vi "FRC.vi"(0 "System no.":i32=1 min=1 max=4 step=1, 1 "Base routine name":string, 2 "Routines to couple to":string[](array[string]), 4 "Remove routine coupling?":bool, 5 "error in":errorcluster) -> (19 "error out":errorcluster)   [LabVIEW 2020]
doc: "Set fast alignment routine coupling: \nIf coupling should be removed, \"Routines to couple to\" has to be 0 or \"Remove routine coupling\" has to be TRUE.\n\nC-887, E-712:"
panel:
  # "Sets Fast alignment Routine Coupling."
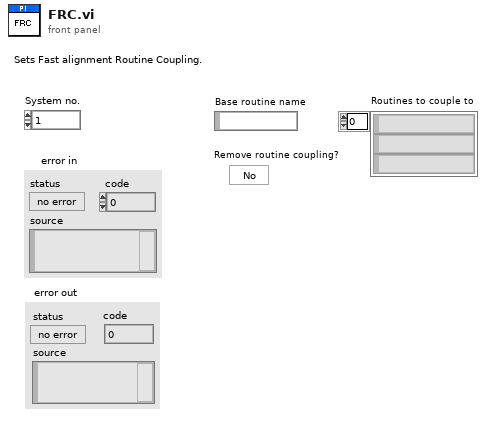
[diagram p1: front panel]
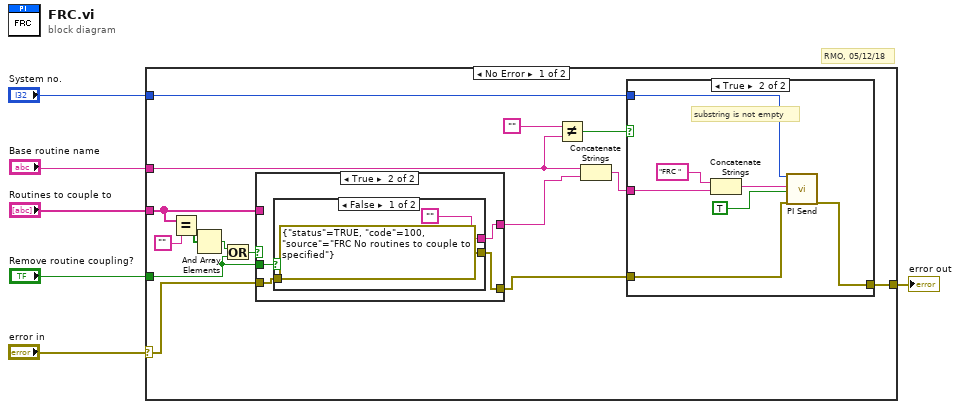
[diagram p0: block diagram]
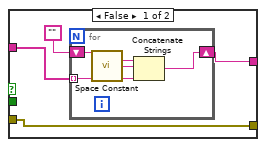
[diagram p2: hidden frame]
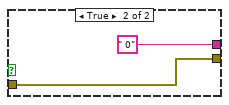
[diagram p3: hidden frame]
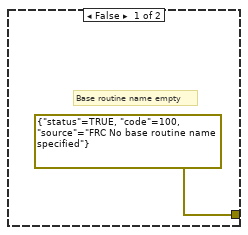
[diagram p4: hidden frame]
diagram:
  # "RMO, 05/12/18"
  n1 = case shown="No Error" "error in" {
    selector: "error in" -> [w7 w46]
    tunnel: [w21 w46] -> w6
    tunnel: "System no." -> [w20 _]
    tunnel: "Base routine name" -> [w18 _]
    tunnel: "Remove routine coupling?" -> [w8 _]
    tunnel: "Routines to couple to" -> [w15 _]
    frame No Error {
      n2 = Equal?(x=w15, y="") -> (x = y?=w13:bool[])
      n3 = And Array Elements(Boolean array=w13) -> (logical AND=w12:bool)
      n4 = Or(x=w12, y=w8) -> (x .or. y?=w11:bool)
      n5 = case shown="True" w11 {
        tunnel: [w23 w32] -> w17
        tunnel: w15 -> [w25 _]
        tunnel: w7 -> [w22 w30]
        tunnel: [w22 w31] -> w9
        tunnel: w8 -> [_ w33]
        frame False {
          n6 = for {
            tunnel: w25 -> [w28] mode=indexing
            shift-right: [w27] -> w23
            shift-left: "" -> [w26]
            n7 = call "Space Constant.vi"() -> ("String"=w29:string)
            n8 = Concatenate Strings(w26, w29, w28) -> (w27:string)
          }
        }
        frame True {
          n9 = case shown="False" w33 {
            tunnel: ["" " 0"] -> w32
            tunnel: [errorcluster {"status"=TRUE, "code"=100, "source"="FRC No routines to couple to specified"} ("error out") w36] -> w31
            tunnel: w30 -> [_ w36]
            frame False {
            }
            frame True {
            }
          }
        }
      }
      n10 = Not Equal?(x="" ("y"), y=w18) -> (x != y?=w10:bool)
      n11 = Concatenate Strings(w18, w17) -> (w19:string)
      n12 = case shown="True" w10 {
        tunnel: [errorcluster {"status"=TRUE, "code"=100, "source"="FRC No base routine name specified"} ("error out") w42] -> w21
        tunnel: w20 -> [_ w41]
        tunnel: w19 -> [_ w40]
        tunnel: w9 -> [_ w39]
        frame False {
          # "Base routine name empty"
        }
        frame True {
          # "substring is not empty"
          n13 = Concatenate Strings("FRC ", w40) -> (w43:string)
          n14 = call "PI Send.vi"("System no."=w41, "String to send"=w43, "Attach termination char.?"=TRUE ("Attach Linefeed?"), "error in"=w39) -> ("error out"=w42:errorcluster)  [unwired: 2 in, 13 out]
        }
      }
    }
    frame Error {
    }
  }
  "error out" <- w6
